vi "svx_Timebase SC Menu.vi"(6 "Run Mode?":bool, 7 "State":T1={"X Scale"={"Name"="Time", "FString"="%#.2g", "Major Color"=16777238, "Minor Color"=16777216, "Grid Style"=1, "Maximum"=0.5, "Minimum"=0.0, "Autoscale"=TRUE, "Show Scale Label"={"Probe X"=FALSE, "Probe Y"=TRUE}, "Show Scale"={"Probe X"=TRUE, "Probe Y"=TRUE}, "Autoscale Once"=FALSE}, "Y Scale"={"Name"="Amplitude", "FString"="%#.2g", "Major Color"=16777238, "Minor Color"=16777216, "Scale Visible"=TRUE, " Label Visible"=TRUE, "Grid Style"=1, "Autoscale"=TRUE, "Maximum"={"Probe X"=1.0, "Probe Y"=1.0}, "Minimum"={"Probe X"=-1.0, "Probe Y"=-1.0}, "Autoscale Once"=FALSE}, "Plot"={"Point Style"=0, "Line Width"=0, "Line Style"=0, "Plot Color"=16860, "Point/fill"=16860}, "Tacho Point Color"=16711680, "Property Name"=[], "Container Bounds"={"Width"=640, "Height"=360}, "Background color"=16777226, "Legend Visible"=TRUE, "Scale Range Change"=refnum, "Strings[]"={"Custom pair name"=FALSE, "Row Strings []"=[], "Column Strings []"=[]}, "Cursor"={"Cursor Point Style"=13, "Cursor Style"=5, "Cursor Line Width"=1, "Cursor Line Style"=0, "Cursor Color"=16860, "Cursor Name Visible"=TRUE, "Cursor Visible"=TRUE, "Cursor Lock"=FALSE, "Cursor Index"=0}, "Index"=[], "Legend Width"=200, " Parents Tags"=[], "Children Tags"=[], "Open?"=[], "Label"="Timebase Plot", "Cursor X Pos"={"X"=0.0, "Y"=0.0}, "Cursor Y Pos"={"X"=0.0, "Y"=0.0}, "Graph Type"=enum."Probe X and Y", "Prev Graph Type"=enum."Probe X and Y", "Prev Legend Visible"=TRUE, "Cursor Release"=refnum, "Pair Strings Changed?"=FALSE, "Cursor ID"=refnum, "Legend Background"=16777226, "Legend Font"=16777222, "Probe Y Label"="Probe Y", "Probe X Label"="Probe X", "Probe X Label Visible"=TRUE, "Probe Y Label Visible"=TRUE, "Tree Item Width"=200, "# Custom RowStr"=0, "# Custom ColStr"=0, "Property Name"=refnum, "Data Related State"=refnum}, 10 "Refnum":refnum<vi>, 11 "MenuRef":refnum<k9>) -> ()   [LabVIEW 2017, in "SVX Timebase.xctl"]
uses:
  <vilib>/addons/_XControls/Timebase Plot/SVX Timebase.xctl
  <vilib>/addons/_XControls/Timebase Plot/subVIs/svx_Timebase State.ctl
  <vilib>/addons/_XControls/Timebase Plot/subVIs/svx_Timebase Bounds.ctl
  <vilib>/addons/_XControls/Timebase Plot/subVIs/svx_Timebase Graph Types.ctl
  <vilib>/addons/_XControls/Timebase Plot/subVIs/svx_Timebase Data Related State.ctl
panel:
  in  "Run-time\nnew menu":T5(array[cluster])=[{"menu tag"="APP_SC_VISIBLE_ITEMS", "item names"="Plot Legend", "item tags"="USER_SC_SELECTOR", ""}, {"menu tag"="APP_SC_VISIBLE_ITEMS", "item names"="-", "item tags"="APP_SC_SEPERATOR", "USER_SC_SELECTOR"}, {"menu tag"="APP_SC_VISIBLE_ITEMS", "item names"="X Scale", "item tags"="USER_SC_X_SCALE", "APP_SC_SEPERATOR"}, {"menu tag"="APP_SC_VISIBLE_ITEMS", "item names"="Y Scale", "item tags"="USER_SC_Y_SCALE", "USER_SC_X_SCALE"}, {"menu tag"="APP_SC_VISIBLE_ITEMS", "item names"="-", "item tags"="APP_SC_SEPERATOR_2", "USER_SC_Y_SCALE"}, {"menu tag"="APP_SC_VISIBLE_ITEMS", "item names"="Cursor", "item tags"="USER_SC_CURSOR", "APP_SC_SEPERATOR_2"}, {"menu tag"="APP_SC_VISIBLE_ITEMS", "item names"="Cursor Info", "item tags"="USER_SC_CURSOR_INFO", "USER_SC_CURSOR"}, {"menu tag"="APP_SC_VISIBLE_ITEMS", "item names"="Lock Cursor Info Position", "item tags"="USER_SC_LOCK", "USER_SC_CURSOR_INFO"}, {"menu tag"="", "item names"="AutoScale X", "item tags"="USER_SC_AUTOSCALE_X", ""}, {"menu tag"="", "item names"="AutoScale Y", "item tags"="USER_SC_AUTOSCALE_Y", "USER_SC_AUTOSCALE_X"}, {"menu tag"="", "item names"="-", "item tags"="APP_SC_SEPERATOR_3", "USER_SC_AUTOSCALE_Y"}, {"menu tag"="", "item names"="Graph Type", "item tags"="USER_SC_GRAPH_TYPE", "APP_SC_SEPERATOR_3"}, {"menu tag"="USER_SC_GRAPH_TYPE", "item names"="Probe X Only", "item tags"="USER_SC_SHOW_X", ""}, {"menu tag"="USER_SC_GRAPH_TYPE", "item names"="Probe Y Only", "item tags"="USER_SC_SHOW_Y", "USER_SC_SHOW_X"}, {"menu tag"="USER_SC_GRAPH_TYPE", "item names"="Probe X and Y", "item tags"="USER_SC_SHOW_XY", "USER_SC_SHOW_Y"}, {"menu tag"="USER_SC_X_SCALE", "item names"="Probe X", "item tags"="USER_SC_X_SCALE_PROBEX", ""}, {"menu tag"="USER_SC_X_SCALE", "item names"="Probe Y", "item tags"="USER_SC_X_SCALE_PROBEY", "USER_SC_X_SCALE_PROBEX"}]
  in  "Edit-time\nnew menu":T5(array[cluster])=[{"menu tag"="USER_SC_VISIBLE_ITEMS", "item names"="Label", "item tags"="USER_SC_LABEL", ""}, {"menu tag"="USER_SC_VISIBLE_ITEMS", "item names"="Caption", "item tags"="USER_SC_CAPTION", "USER_SC_LABEL"}, {"menu tag"="USER_SC_VISIBLE_ITEMS", "item names"="-", "item tags"="APP_SC_SEPERATOR", "USER_SC_CAPTION"}, {"menu tag"="USER_SC_VISIBLE_ITEMS", "item names"="Plot Legend", "item tags"="USER_SC_SELECTOR", "APP_SC_SEPERATOR"}, {"menu tag"="USER_SC_VISIBLE_ITEMS", "item names"="-", "item tags"="APP_SC_SEPERATOR_2", "USER_SC_SELECTOR"}, {"menu tag"="USER_SC_VISIBLE_ITEMS", "item names"="X Scale", "item tags"="USER_SC_X_SCALE", "APP_SC_SEPERATOR_2"}, {"menu tag"="USER_SC_VISIBLE_ITEMS", "item names"="Y Scale", "item tags"="USER_SC_Y_SCALE", "USER_SC_X_SCALE"}, {"menu tag"="USER_SC_VISIBLE_ITEMS", "item names"="-", "item tags"="APP_SC_SEPERATOR_3", "USER_SC_Y_SCALE"}, {"menu tag"="USER_SC_VISIBLE_ITEMS", "item names"="Cursor", "item tags"="USER_SC_CURSOR", "APP_SC_SEPERATOR_3"}, {"menu tag"="USER_SC_VISIBLE_ITEMS", "item names"="Cursor Info", "item tags"="USER_SC_CURSOR_INFO", "USER_SC_CURSOR"}, {"menu tag"="USER_SC_VISIBLE_ITEMS", "item names"="Lock Cursor Info Position", "item tags"="USER_SC_LOCK", "USER_SC_CURSOR_INFO"}, {"menu tag"="", "item names"="AutoScale X", "item tags"="USER_SC_AUTOSCALE_X", ""}, {"menu tag"="", "item names"="AutoScale Y", "item tags"="USER_SC_AUTOSCALE_Y", "USER_SC_AUTOSCALE_X"}, {"menu tag"="", "item names"="-", "item tags"="APP_SC_SEPERATOR_4", "USER_SC_AUTOSCALE_Y"}, {"menu tag"="", "item names"="Graph Type", "item tags"="USER_SC_GRAPH_TYPE", "APP_SC_SEPERATOR_4"}, {"menu tag"="USER_SC_GRAPH_TYPE", "item names"="Probe X Only", "item tags"="USER_SC_SHOW_X", ""}, {"menu tag"="USER_SC_GRAPH_TYPE", "item names"="Probe Y Only", "item tags"="USER_SC_SHOW_Y", "USER_SC_SHOW_X"}, {"menu tag"="USER_SC_GRAPH_TYPE", "item names"="Probe X and Y", "item tags"="USER_SC_SHOW_XY", "USER_SC_SHOW_Y"}, {"menu tag"="", "item names"="-", "item tags"="APP_SC_SEPERATOR_5", "USER_SC_GRAPH_TYPE"}, {"menu tag"="", "item names"="Properties", "item tags"="USER_SC_PROPERTIES", "APP_SC_SEPARATOR_5"}, {"menu tag"="USER_SC_X_SCALE", "item names"="Probe X", "item tags"="USER_SC_X_SCALE_PROBEX", ""}, {"menu tag"="USER_SC_X_SCALE", "item names"="Probe Y", "item tags"="USER_SC_X_SCALE_PROBEY", "USER_SC_X_SCALE_PROBEX"}]
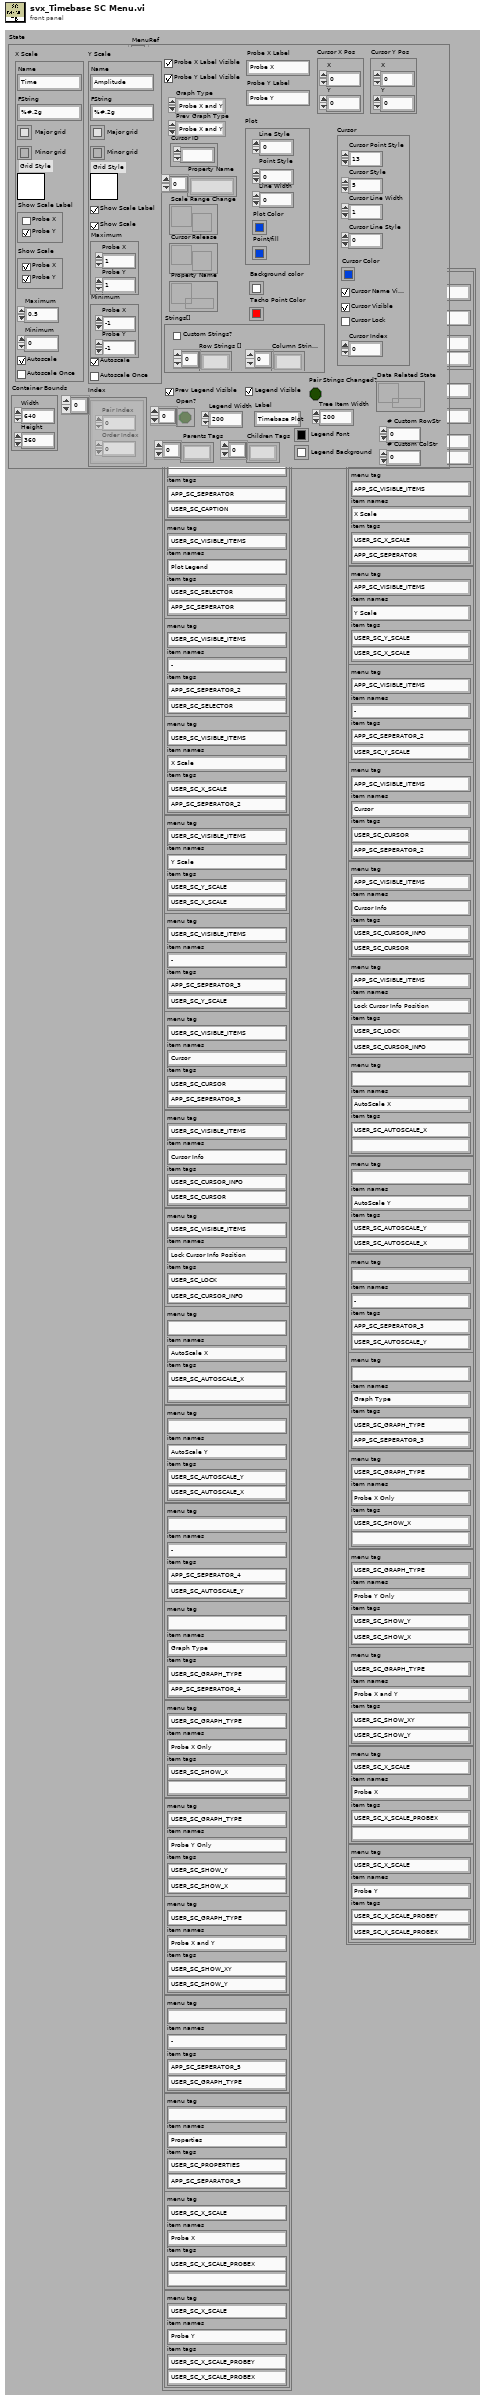
[diagram p1: front panel]
types:
  T1 = typedef "SVX Timebase.xctl/svx_Timebase State.ctl" = cluster{"X Scale":cluster{"Name":string, "FString":string, "Major Color":u32, "Minor Color":u32, "Grid Style":u16, "Maximum":dbl, "Minimum":dbl, "Autoscale":bool, "Show Scale Label":cluster{"Probe X":bool, "Probe Y":bool}, "Show Scale":cluster{"Probe X":bool, "Probe Y":bool}, "Autoscale Once":bool}, "Y Scale":cluster{"Name":string, "FString":string, "Major Color":u32, "Minor Color":u32, "Scale Visible":bool, " Label Visible":bool, "Grid Style":u16, "Autoscale":bool, "Maximum":cluster{"Probe X":dbl, "Probe Y":dbl}, "Minimum":cluster{"Probe X":dbl, "Probe Y":dbl}, "Autoscale Once":bool}, "Plot":cluster{"Point Style":u8, "Line Width":u8, "Line Style":u8, "Plot Color":u32, "Point/fill":u32}, "Tacho Point Color":u32, "Property Name":string[], "Container Bounds":T2, "Background color":u32, "Legend Visible":bool, "Scale Range Change":refnum<user-event>, "Strings[]":cluster{"Custom pair name":bool, "Row Strings []":string[], "Column Strings []":string[]}, "Cursor":cluster{"Cursor Point Style":u8, "Cursor Style":u8, "Cursor Line Width":u8, "Cursor Line Style":u8, "Cursor Color":u32, "Cursor Name Visible":bool, "Cursor Visible":bool, "Cursor Lock":bool, "Cursor Index":i32}, "Index":cluster{"Pair Index":u32, "Order Index":u32}[], "Legend Width":u32, " Parents Tags":string[], "Children Tags":string[], "Open?":bool[], "Label":string, "Cursor X Pos":cluster{"X":dbl, "Y":dbl}, "Cursor Y Pos":cluster{"X":dbl, "Y":dbl}, "Graph Type":T3, "Prev Graph Type":T3, "Prev Legend Visible":bool, "Cursor Release":refnum<user-event>, "Pair Strings Changed?":bool, "Cursor ID":refnum<k1>, "Legend Background":u32, "Legend Font":u32, "Probe Y Label":string, "Probe X Label":string, "Probe X Label Visible":bool, "Probe Y Label Visible":bool, "Tree Item Width":u32, "# Custom RowStr":u32, "# Custom ColStr":u32, "Property Name":refnum<queue>, "Data Related State":T4}
  T2 = typedef "SVX Timebase.xctl/svx_Timebase Bounds.ctl" = cluster{"Width":u32, "Height":u32}
  T3 = typedef "SVX Timebase.xctl/svx_Timebase Graph Types.ctl" = enum16{"Probe X", "Probe Y", "Probe X and Y"}
  T4 = typedef "SVX Timebase.xctl/svx_Timebase Data Related State.ctl" = refnum<queue>
  T5 = cluster{"menu tag":string, "item names":string, "item tags":string, string}[]
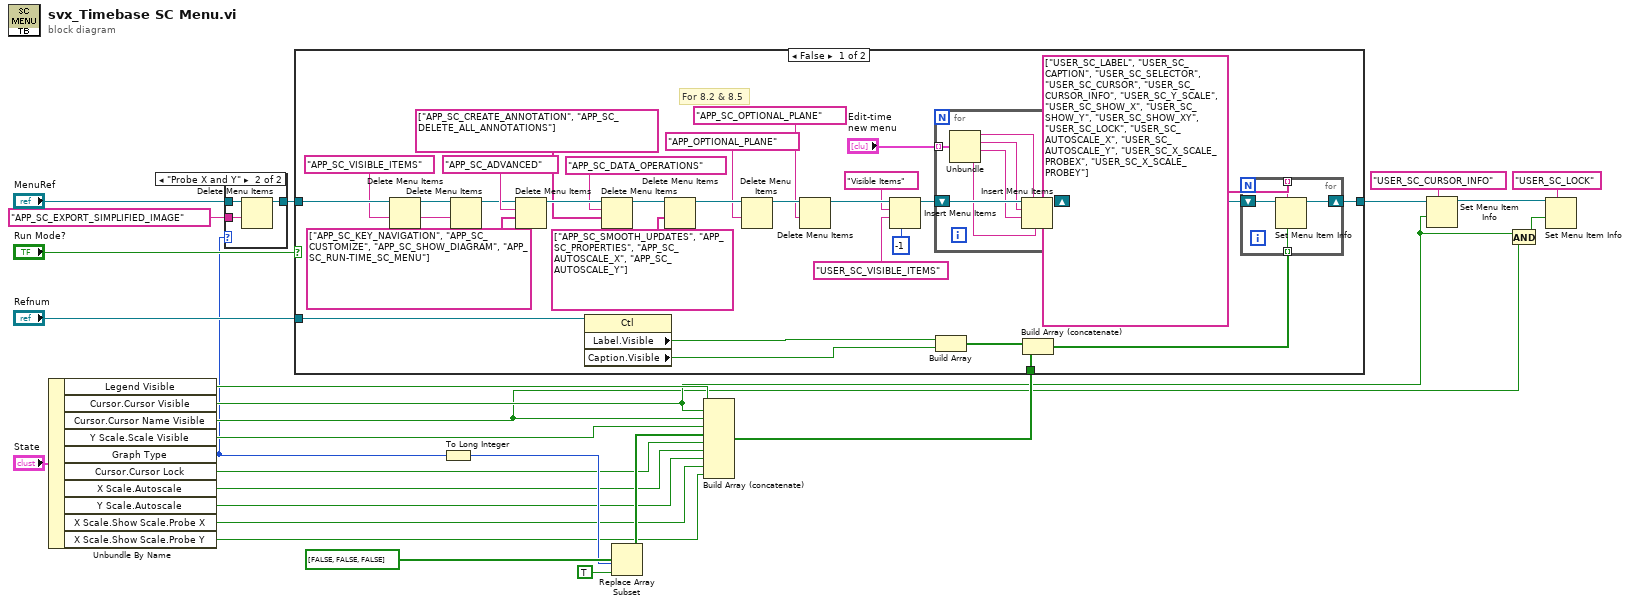
[diagram p0: block diagram]
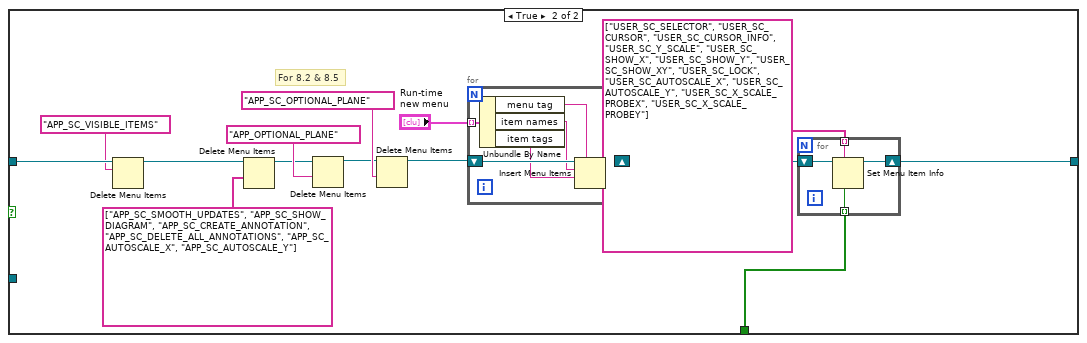
[diagram p3: hidden frame]
diagram:
  n1 = Unbundle By Name("State") -> ("Legend Visible"=w13:bool, "Cursor.Cursor Visible"=w8:bool, "Cursor.Cursor Name Visible"=w7:bool, "Y Scale.Scale Visible"=w24:bool, "Graph Type"=w4:T3, "Cursor.Cursor Lock"=w16:bool, "X Scale.Autoscale"=w15:bool, "Y Scale.Autoscale"=w14:bool, "X Scale.Show Scale.Probe X"=w6:bool, "X Scale.Show Scale.Probe Y"=w5:bool)
  n2 = case shown="\"Probe X and Y\"" w4 {
    tunnel: "MenuRef" -> [w27 w30]
    tunnel: [w27 w29] -> w2
    tunnel: "APP_SC_EXPORT_SIMPLIFIED_IMAGE" ("menu tag") -> [_ w28]
    frame Default {
    }
    frame "Probe X and Y" {
      n3 = Delete Menu Items(7:w28, 9:w30) -> (3:w29:refnum<k9>)  [unwired: 2 in, 1 out]
    }
  }
  n4 = To Long Integer(number=w4) -> (32bit integer=w19:i32)
  n5 = Replace Array Subset(array=bool[] [FALSE, FALSE, FALSE], new element=TRUE, index=w19) -> (w17:bool[])
  n6 = Build Array (concatenate)(w13, w8, w7, w24, w17, w16, w15, w14, w6, w5) -> (w23:bool[])
  n7 = case shown="False" "Run Mode?" {
    tunnel: w2 -> [w56 w85]
    tunnel: "Refnum" -> [w45 _]
    tunnel: w23 -> [w41 w78]
    tunnel: [w35 w77] -> w11
    frame False {
      w53 = "APP_SC_VISIBLE_ITEMS" ("menu tag")
      # "For 8.2 & 8.5"
      n8 = Delete Menu Items(7:w53, 9:w56) -> (3:w55:refnum<k9>)  [unwired: 2 in, 1 out]
      n9 = Delete Menu Items(7:w53, 9:w55) -> (3:w54:refnum<k9>)  [unwired: 2 in, 1 out]
      n10 = Delete Menu Items(7:string[] ["APP_SC_KEY_NAVIGATION", "APP_SC_CUSTOMIZE", "APP_SC_SHOW_DIAGRAM", "APP_SC_RUN-TIME_SC_MENU"], 8:"APP_SC_ADVANCED" ("menu tag"), 9:w54) -> (3:w39:refnum<k9>)  [unwired: 1 in, 1 out]
      n11 = property class="Ctl"(reference=w45) -> ("Label.Visible"=w44:bool, "Caption.Visible"=w43:bool)  [unwired: 1 in, 2 out]
      n12 = Delete Menu Items(7:string[] ["APP_SC_CREATE_ANNOTATION", "APP_SC_DELETE_ALL_ANNOTATIONS"], 8:"APP_SC_DATA_OPERATIONS" ("menu tag"), 9:w39) -> (3:w37:refnum<k9>)  [unwired: 1 in, 1 out]
      n13 = Delete Menu Items(7:string[] ["APP_SC_SMOOTH_UPDATES", "APP_SC_PROPERTIES", "APP_SC_AUTOSCALE_X", "APP_SC_AUTOSCALE_Y"], 9:w37) -> (3:w34:refnum<k9>)  [unwired: 2 in, 1 out]
      n14 = Delete Menu Items(7:"APP_OPTIONAL_PLANE" ("menu tag"), 9:w34) -> (3:w33:refnum<k9>)  [unwired: 2 in, 1 out]
      n15 = Delete Menu Items(7:"APP_SC_OPTIONAL_PLANE" ("menu tag"), 9:w33) -> (3:w52:refnum<k9>)  [unwired: 2 in, 1 out]
      n16 = Insert Menu Items(4:-1, 7:"USER_SC_VISIBLE_ITEMS", 8:"Visible Items" ("item names"), 9:w52) -> (3:w48:refnum<k9>)  [unwired: 2 in, 2 out]
      n17 = for {
        shift-right: [w70] -> w47
        shift-left: w48 -> [w71]
        tunnel: "Edit-time\nnew menu" -> [w69] mode=indexing
        n18 = Unbundle(w69) -> ("menu tag"=w68:string, "item names"=w67:string, "item tags"=w66:string, w65:string)
        n19 = Insert Menu Items(4:w65, 5:w68, 7:w66, 8:w67, 9:w71) -> (3:w70:refnum<k9>)  [unwired: 1 in, 2 out]
      }
      n20 = Build Array(w44, w43) -> (w42:bool[])
      n21 = Build Array (concatenate)(w42, w41) -> (w40:bool[])
      n22 = for {
        shift-right: [w63] -> w35
        shift-left: w47 -> [w64]
        tunnel: string[] ["USER_SC_LABEL", "USER_SC_CAPTION", "USER_SC_SELECTOR", "USER_SC_CURSOR", "USER_SC_CURSOR_INFO", "USER_SC_Y_SCALE", "USER_SC_SHOW_X", "USER_SC_SHOW_Y", "USER_SC_SHOW_XY", "USER_SC_LOCK", "USER_SC_AUTOSCALE_X", "USER_SC_AUTOSCALE_Y", "USER_SC_X_SCALE_PROBEX", "USER_SC_X_SCALE_PROBEY"] ("item tags") -> [w62] mode=indexing
        tunnel: w40 -> [w61] mode=indexing
        n23 = Set Menu Item Info(6:w61, 7:w62, 11:w64) -> (3:w63:refnum<k9>)  [unwired: 4 in, 1 out]
      }
    }
    frame True {
      # "For 8.2 & 8.5"
      n24 = Delete Menu Items(8:"APP_SC_VISIBLE_ITEMS" ("menu tag"), 9:w85) -> (3:w84:refnum<k9>)  [unwired: 2 in, 1 out]
      n25 = Delete Menu Items(7:string[] ["APP_SC_SMOOTH_UPDATES", "APP_SC_SHOW_DIAGRAM", "APP_SC_CREATE_ANNOTATION", "APP_SC_DELETE_ALL_ANNOTATIONS", "APP_SC_AUTOSCALE_X", "APP_SC_AUTOSCALE_Y"], 9:w84) -> (3:w73:refnum<k9>)  [unwired: 2 in, 1 out]
      n26 = Delete Menu Items(7:"APP_OPTIONAL_PLANE" ("menu tag"), 9:w73) -> (3:w74:refnum<k9>)  [unwired: 2 in, 1 out]
      n27 = Delete Menu Items(7:"APP_SC_OPTIONAL_PLANE" ("menu tag"), 9:w74) -> (3:w72:refnum<k9>)  [unwired: 2 in, 1 out]
      n28 = for {
        tunnel: "Run-time\nnew menu" -> [w94] mode=indexing
        shift-right: [w90] -> w79
        shift-left: w72 -> [w95]
        n29 = Unbundle By Name(w94) -> ("menu tag"=w93:string, "item names"=w92:string, "item tags"=w91:string)
        n30 = Insert Menu Items(5:w93, 7:w91, 8:w92, 9:w95) -> (3:w90:refnum<k9>)  [unwired: 2 in, 2 out]
      }
      n31 = for {
        shift-right: [w88] -> w77
        shift-left: w79 -> [w89]
        tunnel: string[] ["USER_SC_SELECTOR", "USER_SC_CURSOR", "USER_SC_CURSOR_INFO", "USER_SC_Y_SCALE", "USER_SC_SHOW_X", "USER_SC_SHOW_Y", "USER_SC_SHOW_XY", "USER_SC_LOCK", "USER_SC_AUTOSCALE_X", "USER_SC_AUTOSCALE_Y", "USER_SC_X_SCALE_PROBEX", "USER_SC_X_SCALE_PROBEY"] ("item tags") -> [w87] mode=indexing
        tunnel: w78 -> [w86] mode=indexing
        n32 = Set Menu Item Info(6:w86, 7:w87, 11:w89) -> (3:w88:refnum<k9>)  [unwired: 4 in, 1 out]
      }
    }
  }
  n33 = Set Menu Item Info(7:"USER_SC_CURSOR_INFO" ("item tag"), 9:w8, 11:w11) -> (3:w10:refnum<k9>)  [unwired: 4 in, 1 out]
  n34 = And(x=w8, y=w7) -> (x .and. y?=w9:bool)
  n35 = Set Menu Item Info(7:"USER_SC_LOCK" ("item tag"), 9:w9, 11:w10) -> ()  [unwired: 4 in, 2 out]
